vi "Set Cmd.vi"(8 "error in (no error)":errorcluster caption="entrée d'erreur (pas d'erreur)", 10 "CMD":string, 11 "P2056_Send_Command_UART en entrée":refnum<class "P2056_Send_Command_UART.lvclass">) -> (0 "error out":errorcluster caption="sortie d'erreur", 3 "P2056_Send_Command_UART en sortie":refnum<class "P2056_Send_Command_UART.lvclass">)   [LabVIEW 2020, in "Library Test.lvlib" / "P2056_Send_Command_UART.lvclass"]
uses:
  P2056_Send_Command_UART.lvclass
  P2056_Send_Command_UART.lvclass/P2056_Send_Command_UART.ctl
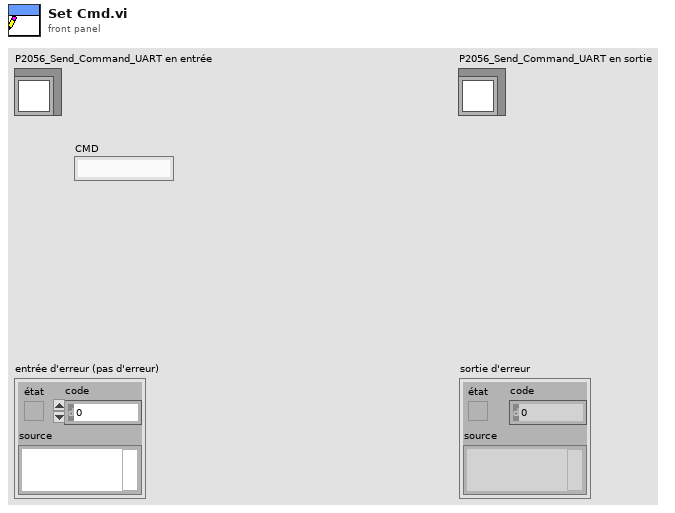
[diagram p1: front panel]
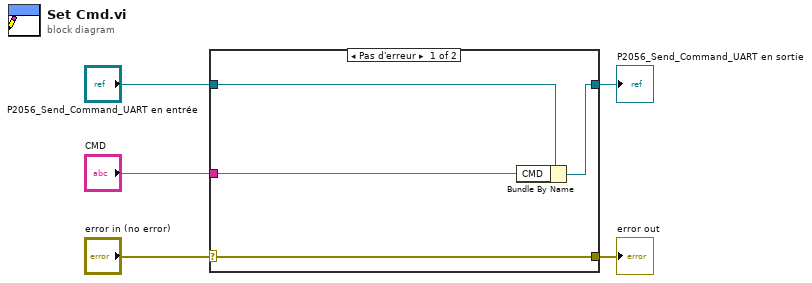
[diagram p0: block diagram]
diagram:
  n1 = case shown="Pas d'erreur" "error in (no error)" {
    selector: "error in (no error)" -> [w9 w10]
    tunnel: [w9 w10] -> w4
    tunnel: [w7 w11] -> w2
    tunnel: "P2056_Send_Command_UART en entrée" -> [w8 w11]
    tunnel: "CMD" -> [w6 _]
    frame No Error {
      n2 = Bundle By Name(cluster=w8, "CMD"=w6) -> (w7:refnum<class "P2056_Send_Command_UART.lvclass">)
    }
    frame Error {
    }
  }
  "error out" <- w4
  "P2056_Send_Command_UART en sortie" <- w2
